vi "toStringArray.vi"(8 "error in (no error)":errorcluster, 11 "PlayFile in":refnum<class "PlayFile.lvclass">) -> (0 "error out":errorcluster, 2 "eventStringArray":string[](array[string]), 3 "PlayFile out":refnum<class "PlayFile.lvclass">)   [LabVIEW 2009, in "Tools.lvlib" / "Scripting.lvlib" / "PlayFile.lvclass"]
uses:
  PlayFile.lvclass
  ScriptEvent.lvclass
  PlayFile.lvclass/PlayFile.ctl
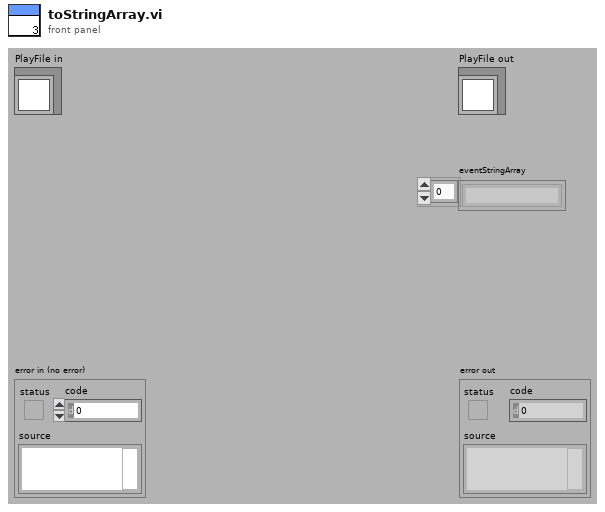
[diagram p1: front panel]
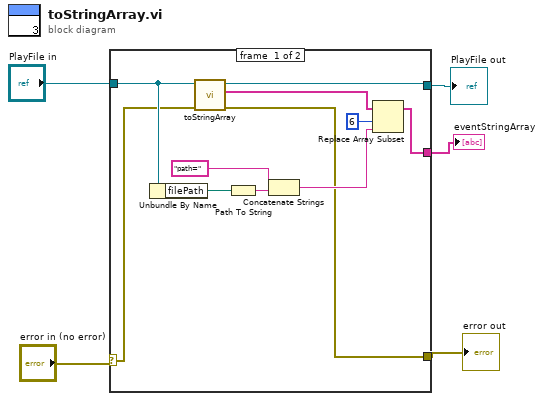
[diagram p0: block diagram]
diagram:
  n1 = case shown="No Error" "error in (no error)" {
    selector: "error in (no error)" -> [w14 w17]
    tunnel: [w6 w17] -> w4
    tunnel: [w16 w18] -> w3
    tunnel: "PlayFile in" -> [w15 w18]
    tunnel: [w7 _] -> w1
    frame #0 {
      n2 = Unbundle By Name(w15) -> ("filePath"=w12:path)
      n3 = call-parent "toStringArray.vi"("error in (no error)"=w14, "ScriptEvent in"=w15) -> ("error out"=w6:errorcluster, "eventStringArray"=w10:string[], "ScriptEvent out"=w16:refnum<class "PlayFile.lvclass">)  [unwired: 7 in]
      n4 = Path To String(path=w12) -> (string=w11:string)
      n5 = Concatenate Strings("path=", w11) -> (w8:string)
      n6 = Replace Array Subset(array=w10, new element=w8, index=6) -> (w7:string[])
    }
    frame #1 {
    }
  }
  "error out" <- w4
  "PlayFile out" <- w3
  "eventStringArray" <- w1
